vi "QD_Main_Module.vi"(0 "Data_In":T1, 1 "Max_Queue_Size_In":i32=-1, 2 "Queue_Name_In":string, 5 "Time_Out_In_ms (-1)":i32, 11 "Error_In":errorcluster, 13 "Queue_Operation":T2=enum."Enqueue") -> (4 "Data_Out":T1, 6 "Total_Data":T1[](array[typedef]), 15 "Error_Out":errorcluster)   [LabVIEW 2023]
doc: "Used to transfer data from one vi to another using queue."
uses:
  Controls/Queue_Operation_Select.ctl
  Controls/State_and_Data.ctl
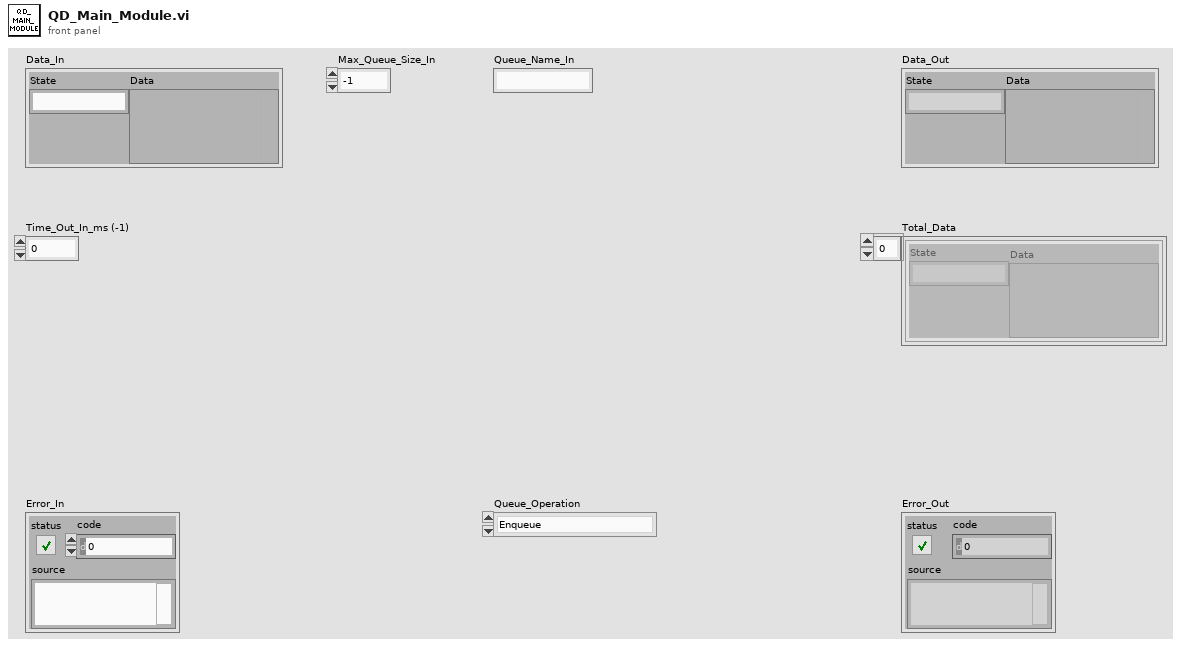
[diagram p1: front panel]
types:
  T1 = typedef "State_and_Data.ctl" = cluster{"State":string, "Data":variant}
  T2 = typedef "Queue_Operation_Select.ctl" = enum16{"Obtain_Queue", "Enqueue", "Enqueue_First", "Enqueue_N", "Lossy_Enqueue", "Preview", "Queue_Status", "Dequeue", "Flush", "Release_Queue"}
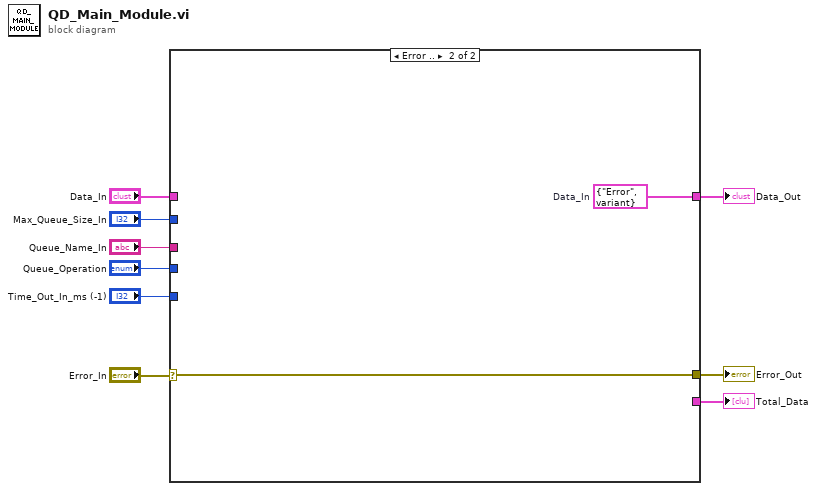
[diagram p0: block diagram]
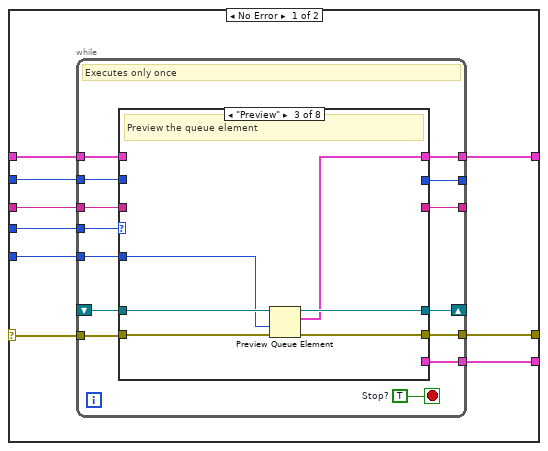
[diagram p2: hidden frame]
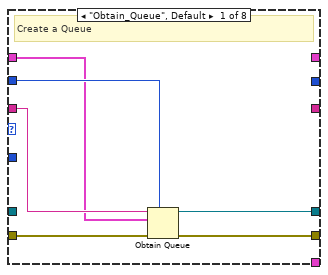
[diagram p3: hidden frame]
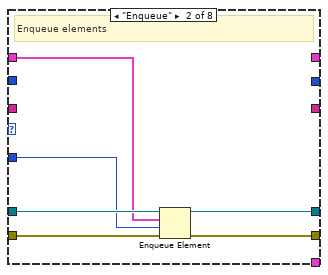
[diagram p4: hidden frame]
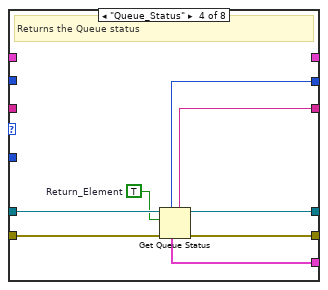
[diagram p5: hidden frame]
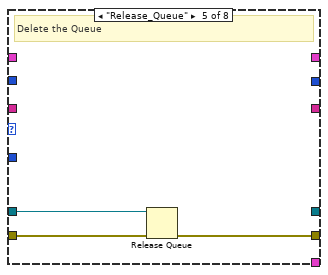
[diagram p6: hidden frame]
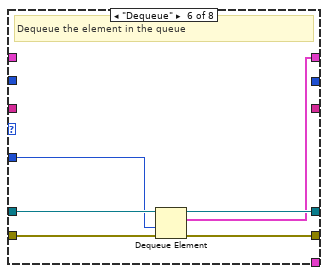
[diagram p7: hidden frame]
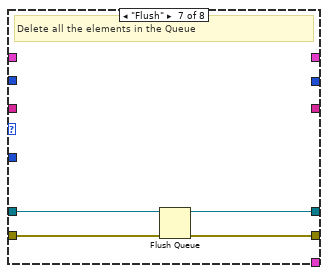
[diagram p8: hidden frame]
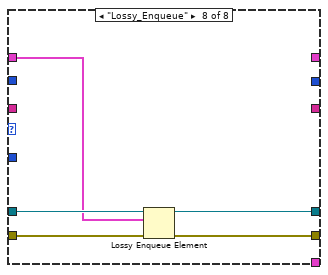
[diagram p9: hidden frame]
diagram:
  n1 = case shown="Error .." "Error_In" {
    selector: "Error_In" -> [w10 w78]
    tunnel: "Max_Queue_Size_In" -> [w18 _]
    tunnel: [w17 w78] -> w8
    tunnel: "Data_In" -> [w16 _]
    tunnel: "Time_Out_In_ms (-1)" -> [w15 _]
    tunnel: [w14 w77] -> w5
    tunnel: "Queue_Operation" -> [w13 _]
    tunnel: "Queue_Name_In" -> [w12 _]
    tunnel: [w11 _] -> w2
    frame No Error {
      n2 = while {
        tunnel: w18 -> [w32]
        tunnel: w15 -> [w29]
        tunnel: [w27] -> _
        tunnel: w13 -> [w24]
        tunnel: [w22] -> w11
        shift-right: [w25] -> _
        shift-left: _ -> [w20]
        tunnel: w10 -> [w21]
        tunnel: [w31] -> w17
        tunnel: w16 -> [w30]
        tunnel: [w28] -> w14
        tunnel: w12 -> [w23]
        tunnel: [w26] -> _
        stop <- w19 stop-if-true
        w19 = TRUE  # Stop?
        # "Executes only once"
        n3 = case shown="\"Preview\"" w24 {
          tunnel: w21 -> [w38 w44 w49 w57 w60 w66 w70 w75]
          tunnel: w23 -> [w36 _ _ _ _ _ _ _]
          tunnel: w32 -> [w35 _ _ _ _ _ _ _]
          tunnel: [w33 w40 w48 w56 _ w65 w69 w74] -> w25
          tunnel: [w37 w43 w47 w55 w59 w63 w68 w73] -> w31
          tunnel: w20 -> [_ w42 w50 w58 w61 w67 w71 w76]
          tunnel: w30 -> [w34 w41 _ _ _ _ _ w72]
          tunnel: w29 -> [_ w39 w46 _ _ w62 _ _]
          tunnel: [_ _ w45 _ _ w64 _ _] -> w28
          tunnel: [_ _ _ w54 _ _ _ _] -> w27
          tunnel: [_ _ _ w53 _ _ _ _] -> w26
          tunnel: [_ _ _ w52 _ _ _ _] -> w22
          frame "Obtain_Queue", Default {
            # "Create a Queue"
            n4 = Obtain Queue(max queue size (-1, unlimited)=w35, name (unnamed)=w36, element data type=w34, error in (no error)=w38) -> (queue out=w33:refnum<queue>, error out=w37:errorcluster)  [unwired: 1 in, 1 out]
          }
          frame "Enqueue" {
            # "Enqueue elements"
            n5 = Enqueue Element(queue=w42, element=w41, timeout in ms (-1)=w39, error in (no error)=w44) -> (queue out=w40:refnum<queue>, error out=w43:errorcluster)  [unwired: 1 out]
          }
          frame "Preview" {
            # "Preview the queue element"
            n6 = Preview Queue Element(queue=w50, timeout in ms (-1)=w46, error in (no error)=w49) -> (queue out=w48:refnum<queue>, element=w45:T1, error out=w47:errorcluster)  [unwired: 1 out]
          }
          frame "Queue_Status" {
            w51 = TRUE  # Return_Element
            # "Returns the Queue status"
            n7 = Get Queue Status(queue=w58, return elements? (F)=w51, error in (no error)=w57) -> (queue out=w56:refnum<queue>, queue name=w53:string, max queue size=w54:i32, error out=w55:errorcluster, elements=w52:T1[])  [unwired: 3 out]
          }
          frame "Release_Queue" {
            # "Delete the Queue"
            n8 = Release Queue(queue=w61, error in (no error)=w60) -> (error out=w59:errorcluster)  [unwired: 1 in, 2 out]
          }
          frame "Dequeue" {
            # "Dequeue the element in the queue"
            n9 = Dequeue Element(queue=w67, timeout in ms (-1)=w62, error in (no error)=w66) -> (queue out=w65:refnum<queue>, element=w64:T1, error out=w63:errorcluster)  [unwired: 1 out]
          }
          frame "Flush" {
            # "Delete all the elements in the Queue"
            n10 = Flush Queue(queue=w71, error in (no error)=w70) -> (queue out=w69:refnum<queue>, error out=w68:errorcluster)  [unwired: 1 out]
          }
          frame "Lossy_Enqueue" {
            n11 = Lossy Enqueue Element(queue=w76, element=w72, error in (no error)=w75) -> (queue out=w74:refnum<queue>, error out=w73:errorcluster)  [unwired: 2 out]
          }
        }
      }
    }
    frame Error {
      w77 = T1 {"State"="Error", "Data"=variant}  # Data_In
    }
  }
  "Error_Out" <- w8
  "Data_Out" <- w5
  "Total_Data" <- w2
